vi "Calculate WL derivative v0.3.vi"(3 "pixel index":dbl=512.0 min=0.0 max=1024.0 format="%.2f", 4 "Current Grating Density":enum16{"150", "300", "600", "1200", "1800"}(ring)=enum."600" caption="Grating Density", 5 "Central Wavelength":dbl=600.0 format="%.2f") -> (1 "Wavelength derivative (out)":dbl=571.2504622529284 format="%.4f")   [LabVIEW 2020]
panel:
  out "Detector Pixel Distance":dbl=27.0 format="%.2f"
  out "beta":dbl=0.03851514953863218 format="%.2f"
  out "alpha":dbl=21.141484850461367 format="%.2f"
  out "Spectrometer Mirror angle":dbl=21.18 format="%.2f"
  out "Spectrometer Focal length":dbl=750.0 format="%.1f"
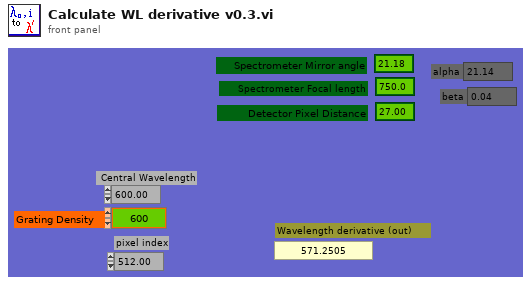
[diagram p1: front panel]
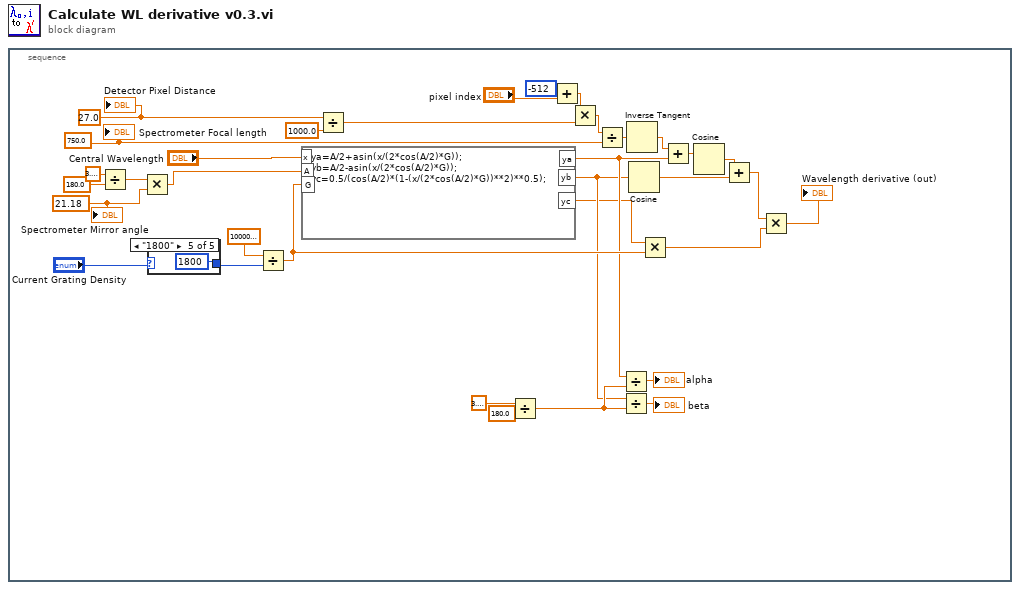
[diagram p0: block diagram]
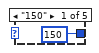
[diagram p2: hidden frame]
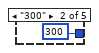
[diagram p3: hidden frame]
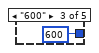
[diagram p4: hidden frame]
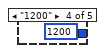
[diagram p5: hidden frame]
diagram:
  n1 = stacked-sequence {
    frame #0 {
      w27 = 21.18 ("Detector Pixel Distance")
      w26 = 750.0 ("Detector Pixel Distance")
      w28 = 27.0 ("x")
      n2 = Divide(x=3.141592653589793, y=180.0) -> (x/y=w20:dbl)
      n3 = Multiply(x=w20, y=w27) -> (x*y=w25:dbl)
      n4 = case shown="\"1800\"" "Current Grating Density" {
        tunnel: [150 300 600 1200 1800] -> w14
        frame "150" {
        }
        frame "300" {
        }
        frame "600" {
        }
        frame "1200" {
        }
        frame "1800" {
        }
      }
      n5 = Divide(x=1000000.0, y=w14) -> (x/y=w24:dbl)
      n6 = formula code="ya=A/2+asin(x/(2*cos(A/2)*G));\nyb=A/2-asin(x/(2*cos(A/2)*G));\nyc=0.5/(cos(A/2)*(1-(x/(2*cos(A/2)*G))**2)**0.5);"("x"="Central Wavelength", "A"=w25, "G"=w24) -> ("ya"=w18:dbl, "yb"=w17:dbl, "yc"=w4:dbl)
      n7 = Divide(x=w28, y=1000.0) -> (x/y=w30:dbl)
      n8 = Divide(x=3.141592653589793, y=180.0) -> (x/y=w23:dbl)
      n9 = Add(x=-512, y="pixel index") -> (x+y=w6:dbl)
      n10 = Multiply(x=w6, y=w30) -> (x*y=w8:dbl)
      n11 = Divide(x=w8, y=w26) -> (x/y=w11:dbl)
      n12 = Divide(x=w18, y=w23) -> (x/y=→"alpha":dbl)
      n13 = Divide(x=w17, y=w23) -> (x/y=→"beta":dbl)
      n14 = Inverse Tangent(1:w11) -> (0:w10:dbl)
      n15 = Cosine(x=w17) -> (cos(x)=w29:dbl)
      n16 = Multiply(x=w4, y=w24) -> (x*y=w3:dbl)
      n17 = Add(x=w10, y=w18) -> (x+y=w9:dbl)
      n18 = Cosine(x=w9) -> (cos(x)=w12:dbl)
      n19 = Add(x=w12, y=w29) -> (x+y=w2:dbl)
      n20 = Multiply(x=w2, y=w3) -> (x*y=→"Wavelength derivative (out)":dbl)
      "Spectrometer Focal length" <- w26
      "Spectrometer Mirror angle" <- w27
      "Detector Pixel Distance" <- w28
    }
  }
